vi "PWM_Write.vi"(8 "error in (no error)":errorcluster, 9 "DC":u8(slide) scale=0.0..255.0, 10 "Pin":u8=4 min=4 max=40, 11 "VISA resource name":refnum<visa-resource-name>) -> (0 "error out":errorcluster, 3 "VISA resource name out":refnum<visa-resource-name>)   [LabVIEW 2025]
doc: "VI que permite hacer una escritura de PWM de 8 bits \nenviando el duty cycle con un valor de 0 a 255"
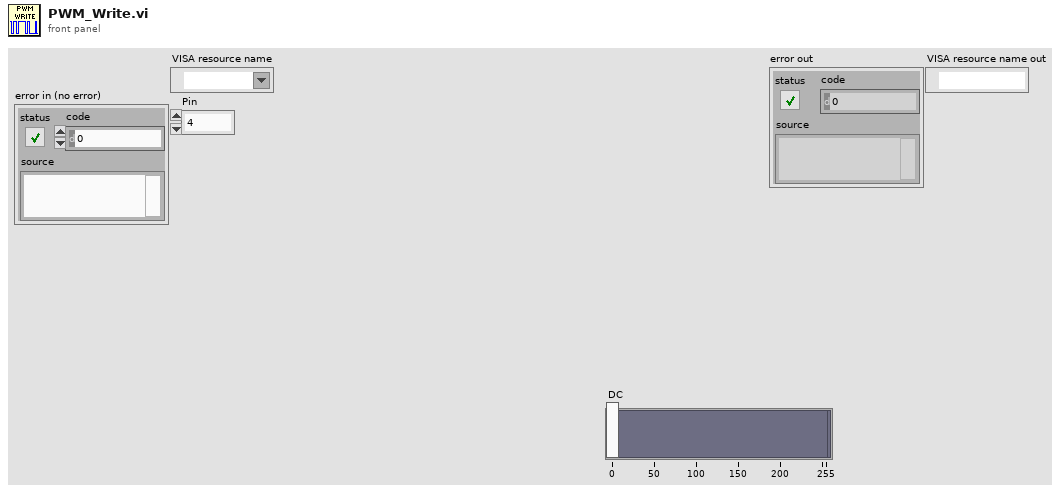
[diagram p1: front panel]
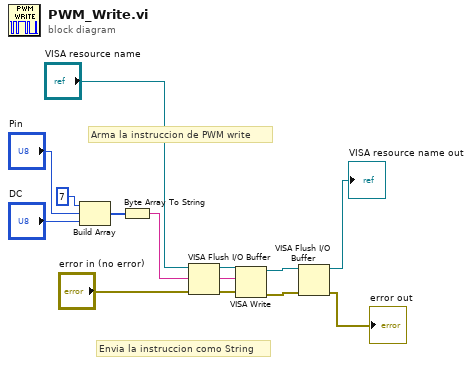
[diagram p0: block diagram]
diagram:
  # "Envia la instruccion como String"
  # "Arma la instruccion de PWM write"
  n1 = Build Array(u8 7, "Pin", "DC") -> (w11:u8[])
  n2 = Byte Array To String(unsigned byte array=w11) -> (string=w13:string)
  n3 = VISA Flush I/O Buffer(VISA resource name="VISA resource name", error in (no error)="error in (no error)") -> (VISA resource name out=w4:refnum<visa-resource-name>, error out=w3:errorcluster)  [unwired: 1 in]
  n4 = VISA Write(VISA resource name=w4, write buffer=w13, error in (no error)=w3) -> (VISA resource name out=w7:refnum<visa-resource-name>, error out=w8:errorcluster)  [unwired: 1 out]
  n5 = VISA Flush I/O Buffer(VISA resource name=w7, error in (no error)=w8) -> (VISA resource name out=→"VISA resource name out":refnum<visa-resource-name>, error out=→"error out":errorcluster)  [unwired: 1 in]
